vi "TestM1M3ILCLoopPerformance.vi"() -> ()   [LabVIEW 2016]
uses:
  Model/Model.lvclass
  Common_RT_Modbus/ModbusBuffer/ModbusBuffer.lvclass
  Model/Model.lvclass/Model.ctl
  ILCCommunications/ILCCommunications.lvclass/ILCCommunications.ctl
  Common_RT_HPILC/HPILC/HPILC.lvclass/HPILC.ctl
  Common_RT_ILC/ILC/ILC.lvclass/ILC.ctl
  Common_RT_Modbus/ModbusBuffer/ModbusBuffer.lvclass/ModbusBuffer.ctl
  ILCCommunications/reportAllHPForceAndStatus.vi
  ILCCommunications/reportAllHPServerStatus.vi
  ILCCommunications/broadcastHPFreezeSensorValues.vi
  ILCCommunications/reportHPForceAndStatus.vi
  ILCCommunications/reportHPServerStatus.vi
  Common_RT_HPILC/HPILC/addBroadcastFreezeSensorValuesFrame.vi
  Common_RT_HPILC/HPILC/createForceAndStatusFrame.vi
  ILCCommunications/reportServerStatus.vi
  Common_RT_Modbus/ModbusBuffer/writeHeader.vi
  Common_RT_Modbus/ModbusBuffer/writeU8.vi
  Common_RT_Modbus/ModbusBuffer/writeCRC.vi
  Common_RT_Modbus/ModbusBuffer/writeDelay.vi
  Common_RT_ILC/ILC/getILCData.vi
  Common_RT_Modbus/ModbusBuffer/writeEndOfFrame.vi
  Common_RT_Modbus/ModbusBuffer/writeWaitForRx.vi
  Common_RT_ILC/ILC/addReportServerStatusFrame.vi
  Common_RT_Modbus/ModbusBuffer/writeByteInstruction.vi
  Common_RT_Modbus/ModbusBuffer/calculateCRC.vi
  Common_RT_HPILC/HPILC/HPILC.lvclass
  D:/Code/ts_M1M3Support/Common_RT_ILC/ILC/ILC.lvclass
panel:
  out "Time (us)":u32
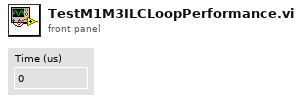
[diagram p1: front panel]
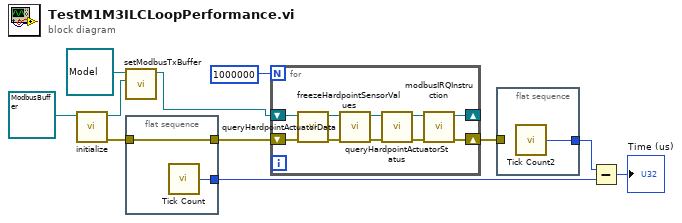
[diagram p0: block diagram]
diagram:
  n1 = call "initialize.vi"("ModbusBuffer in"=refnum<class "ModbusBuffer.lvclass"> refnum ("ModbusTxBuffer")) -> ("error out"=w5:errorcluster, "ModbusBuffer out"=w9:refnum<class "ModbusBuffer.lvclass">)  [unwired: 9 in]
  n2 = call "setModbusTxBuffer.vi"("ModbusTxBuffer"=w9, "Model in"=refnum<class "Model.lvclass"> refnum ("Model.lvclass")) -> ("Model out"=w8:refnum<class "Model.lvclass">)  [unwired: 9 in]
  n3 = flat-sequence {
    tunnel: [w13] -> w6
    tunnel: w5 -> [w13]
    tunnel: [w12] -> w2
    frame #0 {
      n4 = call "Tick Count"() -> ("Tick Count(uSec)"=w12:u32)
    }
  }
  n5 = for {
    N: 1000000 -> [_]
    shift-right: [w15] -> _
    shift-left: w8 -> [w14]
    shift-right: [w16] -> w4
    shift-left: w6 -> [w20]
    n6 = call "freezeHardpointSensorValues.vi"("error in (no error)"=w20, "Model in"=w14) -> ("error out"=w19:errorcluster, "Model out"=w21:refnum<class "Model.lvclass">)  [unwired: 8 in]
    n7 = call "queryHardpointActuatorData.vi"("error in (no error)"=w19, "Model in"=w21) -> ("error out"=w18:errorcluster, "Model out"=w22:refnum<class "Model.lvclass">)  [unwired: 8 in]
    n8 = call "queryHardpointActuatorStatus.vi"("error in (no error)"=w18, "Model in"=w22) -> ("error out"=w17:errorcluster, "Model out"=w23:refnum<class "Model.lvclass">)  [unwired: 8 in]
    n9 = call "modbusIRQInstruction.vi"("error in (no error)"=w17, "Model in"=w23) -> ("error out"=w16:errorcluster, "Model out"=w15:refnum<class "Model.lvclass">)  [unwired: 8 in]
  }
  n10 = flat-sequence {
    tunnel: w4 -> [_]
    tunnel: [w24] -> w3
    frame #0 {
      n11 = call "Tick Count2"() -> ("Tick Count(uSec)"=w24:u32)
    }
  }
  n12 = Subtract(x=w3, y=w2) -> (x-y=→"Time (us)":u32)
